vi "Launch Actor from File Path.vi"(7 "Actor Class":refnum<class "_Parent Actor Template.lvclass">, 8 "error in (no error)":errorcluster, 10 "Actor-to-Caller Enqueuer":refnum<class "Message Enqueuer.lvclass">, 11 "Actor Path":path) -> (0 "error out":errorcluster, 3 "Caller-to-Actor Enqueuer":refnum<class "Message Enqueuer.lvclass">)   [LabVIEW 2016]
doc: "Launches an Actor from a file path and returns its enqueuer."
uses:
  <vilib>/ActorFramework/Message Enqueuer/Message Enqueuer.lvclass
  _Parent Actor Template.lvclass
  C:/Program Files (x86)/National Instruments/LabVIEW 2016/vi.lib/ActorFramework/Actor/Actor.lvclass
  <vilib>/ActorFramework/Actor/Actor.lvclass
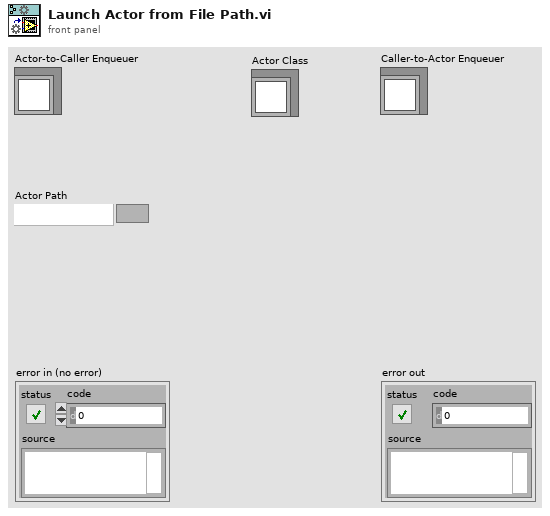
[diagram p1: front panel]
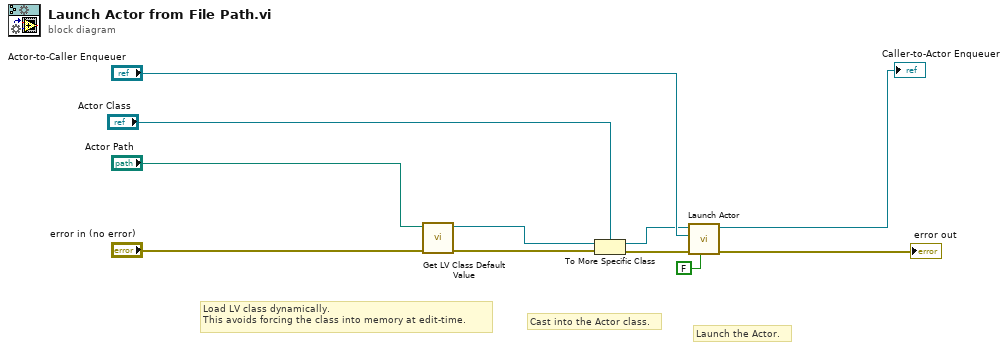
[diagram p0: block diagram]
diagram:
  # "Launch the Actor."
  # "Cast into the Actor class."
  # "Load LV class dynamically.\nThis avoids forcing the class into memory at edit-time."
  n1 = call <vilib>:"Get LV Class Default Value.vi"("error in (no error)"="error in (no error)", "class path"="Actor Path") -> ("error out"=w5:errorcluster, "object"=w4:refnum<class>)  [unwired: 8 in]
  n2 = To More Specific Class(target class="Actor Class", reference=w4, error in=w5) -> (specific class reference=w2:refnum<class "_Parent Actor Template.lvclass">, error out=w3:errorcluster)
  n3 = call <vilib>:"Launch Actor.vi"("Open Actor Core front panel? (F)"=FALSE, "error in (no error)"=w3, "Actor-to-Caller Enqueuer"="Actor-to-Caller Enqueuer", "Actor"=w2) -> ("error out"=→"error out":errorcluster, "Caller-To-Actor Enqueuer"=→"Caller-to-Actor Enqueuer":refnum<class "Message Enqueuer.lvclass">)  [unwired: 6 in]
